vi "Format and write to Excel.vi"(8 "error in (no error)":errorcluster, 10 "Data":cluster{"Position":dbl, "Value":dbl}[](array[cluster]), 11 "selected path":path) -> (0 "error out":errorcluster)   [LabVIEW 2020]
uses:
  <vilib>/Utility/file.llb/Write Delimited Spreadsheet (string).vi
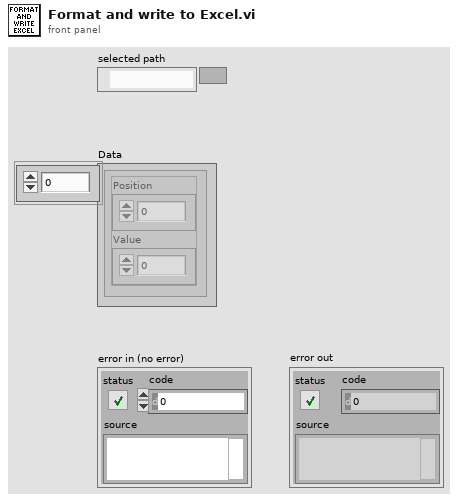
[diagram p1: front panel]
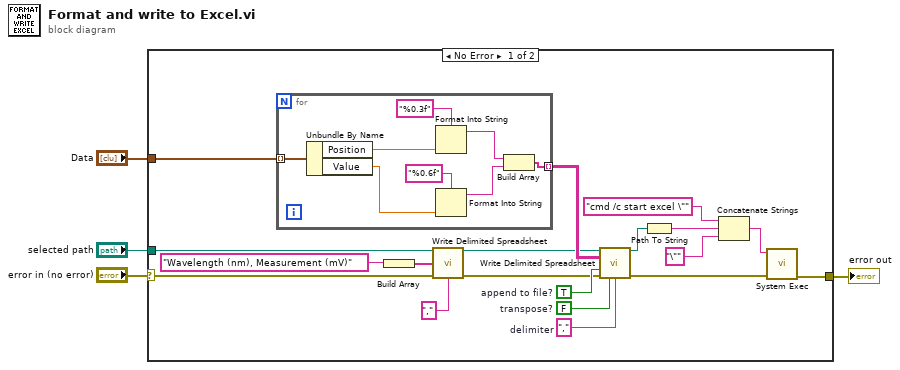
[diagram p0: block diagram]
diagram:
  n1 = case shown="No Error" "error in (no error)" {
    selector: "error in (no error)" -> [w10 w32]
    tunnel: [w13 w32] -> w4
    tunnel: "selected path" -> [w12 _]
    tunnel: "Data" -> [w5 _]
    frame No Error {
      w23 = ","  # delimiter
      w20 = TRUE  # append to file?
      w21 = FALSE  # transpose?
      n2 = for {
        tunnel: [w30] -> w22 mode=indexing
        tunnel: w5 -> [w26] mode=indexing
        n3 = Unbundle By Name(w26) -> ("Position"=w25:dbl, "Value"=w24:dbl)
        n4 = Format Into String(format string="%0.3f" ("format (%.3f)"), w25) -> (resulting string=w28:string)  [unwired: 2 in, 1 out]
        n5 = Format Into String(format string="%0.6f" ("format (%.3f)"), w24) -> (resulting string=w29:string)  [unwired: 2 in, 1 out]
        n6 = Build Array(w28, w29) -> (w30:string[])
      }
      n7 = Build Array("Wavelength (nm), Measurement (mV)") -> (w6:string[])
      n8 = call-poly <vilib>:"Write Delimited Spreadsheet.vi"("file path (dialog if empty)"=w12, "1D data"=w6, "error in (no error)"=w10, "delimiter (\\t)"="," ("delimiter (\\t)")) -> ("new file path (Not A Path if cancelled)"=w11:path, "error out"=w9:errorcluster)  [unwired: 10 in]
      n9 = call-poly <vilib>:"Write Delimited Spreadsheet.vi"("file path (dialog if empty)"=w11, "2D data"=w22, "append to file? (new file:F)"=w20, "error in (no error)"=w9, "transpose? (no:F)"=w21, "delimiter (\\t)"=w23) -> ("new file path (Not A Path if cancelled)"=w18:path, "error out"=w19:errorcluster)  [unwired: 8 in]
      n10 = Path To String(path=w18) -> (string=w15:string)
      n11 = Concatenate Strings("cmd /c start excel \"" ("string"), w15, "\"" ("string")) -> (w17:string)
      n12 = call <vilib>:"System Exec.vi"("error in (no error)"=w19, "command line"=w17) -> ("error out"=w13:errorcluster)  [unwired: 6 in, 3 out]
    }
    frame Error {
    }
  }
  "error out" <- w4
